vi "TB-Check Initializatin Status.vi"(0 "state in":T1, 2 "Starts":refnum<vi>, 11 "error in (no error)":errorcluster) -> (4 "state out":T1, 15 "error out":errorcluster)   [LabVIEW 2020]
uses:
  Typedefs/TB-Runtime state.ctl
  <vilib>/sound2/lvsound2.llb/Sound File Refnum.ctl
  Typedefs/TB-Setup Log.ctl
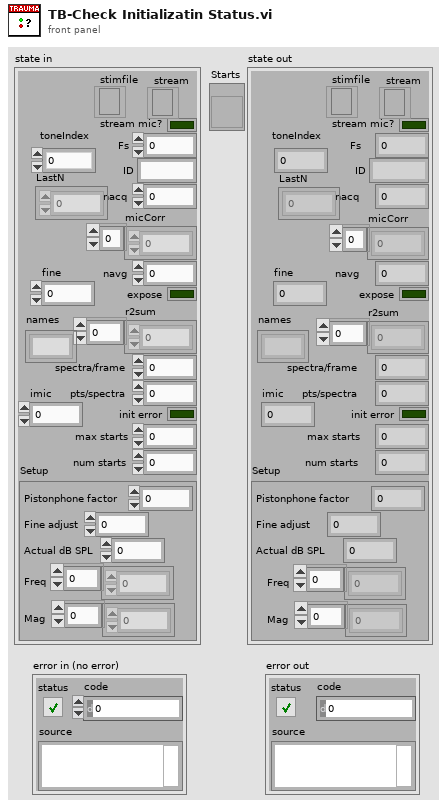
[diagram p1: front panel]
types:
  T1 = typedef "TB-Runtime state.ctl" = cluster{"stimfile":T2, "stream mic?":bool, "Fs":dbl, "ID":string, "micCorr":dbl[], "navg":i32, "r2sum":dbl[], "expose":bool, "spectra/frame":i32, "pts/spectra":i32, "nacq":i32, "init error":bool, "max starts":i32, "num starts":i32, "Setup":T3, "toneIndex":i32, "LastN":dbl[], "fine":dbl, "imic":i32, "stream":refnum<file>, "names":string[]}
  T2 = typedef "Sound File Refnum.ctl" = refnum<file>
  T3 = typedef "TB-Setup Log.ctl" = cluster{"Pistonphone factor":dbl, "Fine adjust":dbl, "Actual dB SPL":dbl, "Freq":dbl[], "Mag":dbl[]}
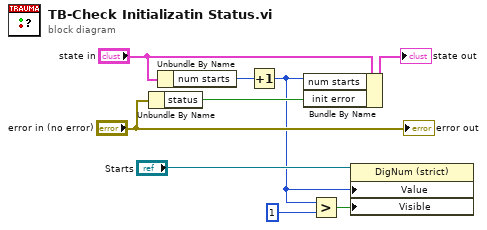
[diagram p0: block diagram]
diagram:
  n1 = Unbundle By Name("error in (no error)") -> ("status"=w8:bool)
  n2 = Unbundle By Name("state in") -> ("num starts"=w5:i32)
  n3 = Increment(x=w5) -> (x+1=w3:i32)
  n4 = Bundle By Name(cluster="state in", "num starts"=w3, "init error"=w8) -> (→"state out":T1)
  n5 = Greater?(x=w3, y=1) -> (0:w1:bool)
  n6 = property class="DigNum (strict)"(reference="Starts", "Value"=w3, "Visible"=w1) -> ()  [unwired: 1 in, 2 out]
  "error out" <- "error in (no error)"
